vi "Status.vi"(8 "error in (no error)":errorcluster, 11 "HotCoil Settings In":T1) -> (0 "error out":errorcluster, 1 "Connection Error":bool, 2 "Running":bool, 3 "HotCoil Settings Out":T1, 4 "Temp":dbl)   [LabVIEW 2021, in "HotCoil.lvlib"]
uses:
  HotCoil.lvlib
  HotCoil Settings.ctl
panel:
  out "in_sp":string[](array[string])
  out "Temperature Array":string[](array[string])
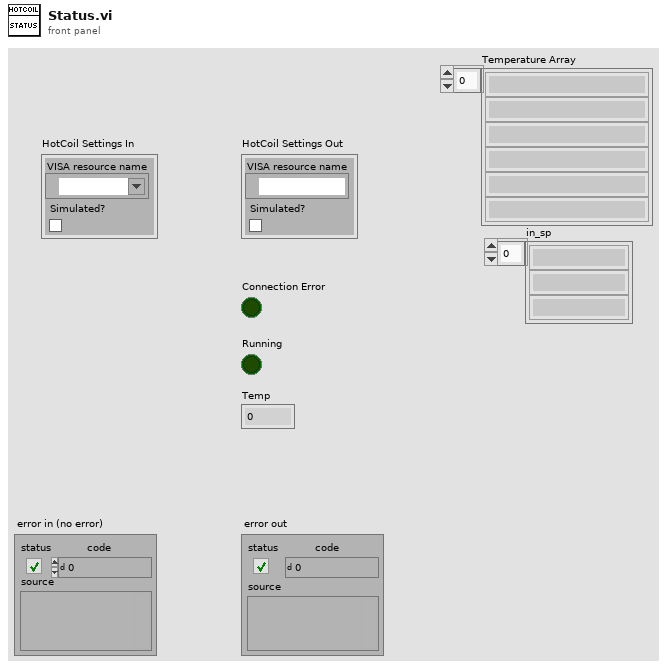
[diagram p1: front panel]
types:
  T1 = typedef "HotCoil.lvlib/HotCoil Settings.ctl" = cluster{"VISA resource name":refnum<visa-resource-name>, "Simulated?":bool}
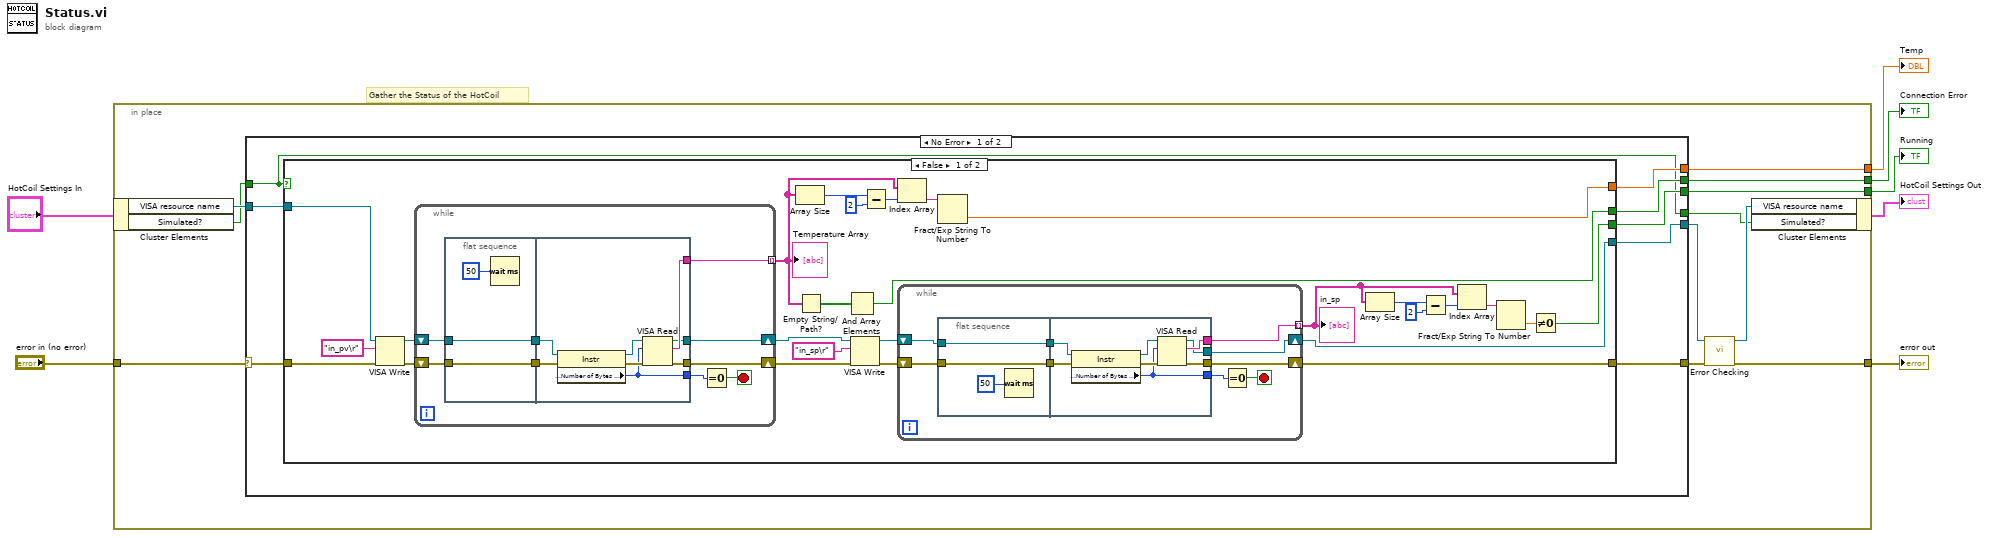
[diagram p0: block diagram]
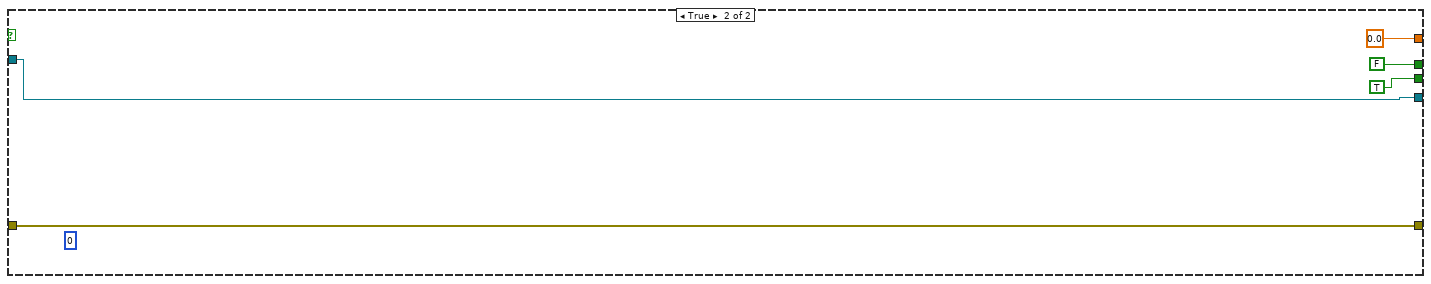
[diagram p2: hidden frame]
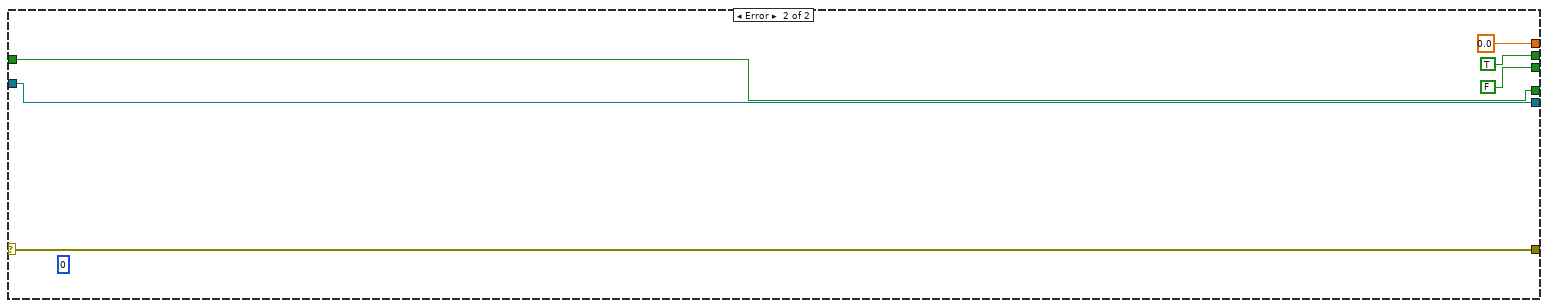
[diagram p3: hidden frame]
diagram:
  # "Gather the Status of the HotCoil"
  n1 = in-place {
    in-place-border: "error in (no error)" -> [w18]
    in-place-border: [w15] -> w6
    in-place-border: [w14] -> w5
    in-place-border: [w13] -> w4
    in-place-border: [w12] -> w3
    n2 = in-place-cluster #1("HotCoil Settings In") -> ("VISA resource name"=w11:refnum<visa-resource-name>, "Simulated?"=w9:bool)
    n3 = case shown="No Error" w18 {
      selector: w18 -> [w26 w104]
      tunnel: [w25 w104] -> w16
      tunnel: [w24 w99] -> w17
      tunnel: [w23 TRUE] -> w14
      tunnel: [w22 FALSE] -> w13
      tunnel: [w21 0.0 ("InternalTemp (out)")] -> w12
      tunnel: w11 -> [w20 w99]
      tunnel: w9 -> [w19 w100]
      tunnel: [w19 w100] -> w8
      frame No Error {
        n4 = case shown="False" w19 {
          tunnel: w26 -> [w52 w98]
          tunnel: [w34 w98] -> w25
          tunnel: [w36 w97] -> w24
          tunnel: w20 -> [w50 w97]
          tunnel: [w46 FALSE] -> w23
          tunnel: [w28 TRUE] -> w22
          tunnel: [w53 0.0 ("InternalTemp (out)")] -> w21
          frame False {
            n5 = VISA Write(VISA resource name=w50, write buffer="in_pv\r", error in (no error)=w52) -> (VISA resource name out=w49:refnum<visa-resource-name>, error out=w48:errorcluster)  [unwired: 1 out]
            n6 = while {
              shift-right: [w82] -> w45
              shift-left: w49 -> [w76]
              shift-right: [w81] -> w44
              shift-left: w48 -> [w75]
              tunnel: [w78] -> w41 mode=indexing
              stop <- w79 stop-if-true
              n7 = flat-sequence {
                tunnel: [w84] -> w77
                tunnel: w76 -> [w84]
                tunnel: w75 -> [w83]
                tunnel: [w83] -> w74
                tunnel: [w93] -> w81
                tunnel: [w92] -> w78
                tunnel: [w91] -> w82
                tunnel: [w88] -> w80
                tunnel: w77 -> [w87]
                tunnel: w74 -> [w86]
                frame #0 {
                  n8 = Wait (ms)(milliseconds to wait=u32 50) -> ()  [unwired: 1 out]
                }
                frame #1 {
                  n9 = property class="Instr"(reference=w87, error in=w86) -> (reference out=w90:refnum<visa-resource-name>, error out=w89:errorcluster, "Serial Settings:Number of Bytes at Serial Port"=w88:u32)
                  n10 = VISA Read(VISA resource name=w90, byte count=w88, error in (no error)=w89) -> (VISA resource name out=w91:refnum<visa-resource-name>, read buffer=w92:string, error out=w93:errorcluster)  [unwired: 1 out]
                }
              }
              n11 = Equal To 0?(x=w80) -> (x = 0?=w79:bool)
            }
            "Temperature Array" <- w41
            n12 = Array Size(array=w41) -> (size(s)=w40:i32)
            n13 = Empty String/Path?(string/path=w41) -> (empty?=w47:bool[])
            n14 = And Array Elements(Boolean array=w47) -> (logical AND=w46:bool)
            n15 = VISA Write(VISA resource name=w45, write buffer="in_sp\r", error in (no error)=w44) -> (VISA resource name out=w37:refnum<visa-resource-name>, error out=w35:errorcluster)  [unwired: 1 out]
            n16 = Subtract(x=w40, y=2) -> (x-y=w42:i32)
            n17 = Index Array(array=w41, index=w42) -> (element=w43:string)
            n18 = while {
              tunnel: [w60] -> w29 mode=indexing
              shift-right: [w62] -> w36
              shift-left: w37 -> [w56]
              shift-right: [w61] -> w34
              shift-left: w35 -> [w54]
              stop <- w59 stop-if-true
              n19 = flat-sequence {
                tunnel: [w64] -> w57
                tunnel: w56 -> [w64]
                tunnel: [w63] -> w55
                tunnel: w54 -> [w63]
                tunnel: [w73] -> w61
                tunnel: [w72] -> w60
                tunnel: [w71] -> w62
                tunnel: [w68] -> w58
                tunnel: w57 -> [w67]
                tunnel: w55 -> [w66]
                frame #0 {
                  n20 = Wait (ms)(milliseconds to wait=u32 50) -> ()  [unwired: 1 out]
                }
                frame #1 {
                  n21 = property class="Instr"(reference=w67, error in=w66) -> (reference out=w70:refnum<visa-resource-name>, error out=w69:errorcluster, "Serial Settings:Number of Bytes at Serial Port"=w68:u32)
                  n22 = VISA Read(VISA resource name=w70, byte count=w68, error in (no error)=w69) -> (VISA resource name out=w71:refnum<visa-resource-name>, read buffer=w72:string, error out=w73:errorcluster)  [unwired: 1 out]
                }
              }
              n23 = Equal To 0?(x=w58) -> (x = 0?=w59:bool)
            }
            "in_sp" <- w29
            n24 = Fract/Exp String To Number(string=w43) -> (number=w53:dbl)  [unwired: 3 in, 1 out]
            n25 = Array Size(array=w29) -> (size(s)=w32:i32)
            n26 = Subtract(x=w32, y=2) -> (x-y=w31:i32)
            n27 = Index Array(array=w29, index=w31) -> (element=w30:string)
            n28 = Fract/Exp String To Number(string=w30) -> (number=w27:dbl)  [unwired: 3 in, 1 out]
            n29 = Not Equal To 0?(x=w27) -> (x != 0?=w28:bool)
          }
          frame True {
            (unwired) u8 0 ("Pumpstage (out)")
          }
        }
      }
      frame Error {
        (unwired) u8 0 ("Pumpstage (out)")
      }
    }
    n30 = call "Error Checking.vi"("error in (no error)"=w16, "VISA resource name"=w17) -> ("error out"=w15:errorcluster, "VISA resource name"=w10:refnum<visa-resource-name>)  [unwired: 7 in, 1 out]
    n31 = in-place-cluster #1("VISA resource name"=w10, "Simulated?"=w8) -> (→"HotCoil Settings Out":T1)
  }
  "error out" <- w6
  "Connection Error" <- w5
  "Running" <- w4
  "Temp" <- w3
